vi "ControllerModels.vi"(9 "Gain in":dbl(slide)=3.0 scale=0.0..10.0, 10 "B":dbl, 11 "A":dbl) -> (3 "Plots":T1={"OpenLoop"=bytes[0], "Gain out"=bytes[146], "CL TF"=bytes[562], "Step Response Graph"=[{"time"=array[396 elements], array[396 elements]}], "Root Locus Graph"=[{[-13.1543317764195, -13.1543317764195], [27.765972114103178, -27.765972114103178]}, {[-26.308663552838997, 0.0], [0.0, 0.0]}, {[], []}, {[-13.154331776419498], [0.0]}, {array[551 elements], array[551 elements]}, {array[551 elements], array[551 elements]}], "Bode Magnitude"=[{"W"=[1.0, 1.0974987654930561, 1.2045035402587823, 1.3219411484660293, 1.45082877849594, 1.5922827933410926, 1.747528400007684, 1.9179102616724888, 2.104904144512021, 2.31012970008316, 2.5353644939701123, 2.7825594022071254, 3.0538555088334163, 3.351602650938843, 3.6783797718286344, 4.037017258596555, 4.430621457583881, 4.862601580065355, 5.33669923120631, 5.857020818056667, 6.428073117284322, 7.054802310718645, 7.742636826811273, 8.497534359086446, 9.326033468832202, 10.235310218990266, 11.23324032978028, 12.328467394420668, 13.530477745798079, 14.84968262254466, 16.297508346206453, 17.88649529057436, 19.63040650040272, 21.54434690031885, 23.644894126454087, 25.950242113997376, 28.480358684358034, 30.996999999999996, 31.257158496882383, 34.30469286314921, 37.64935806792471, 41.3201240011534, 45.34878508128586, 49.77023564332115, 54.62277217684346, 59.94842503189415, 60.99399999999999, 65.79332246575686, 72.20809018385471, 79.2482898353918, 86.97490026177842, 90.99099999999999, 95.4548456661835, 104.76157527896659, 114.9756995397737, 120.98799999999999, 126.18568830660217, 138.48863713938746, 151.99110829529354, 166.81005372000607, 183.07382802953703, 200.92330025650494, 220.51307399030483, 242.0128264794385, 265.608778294669, 291.50530628251806, 319.9267137797388, 351.11917342151366, 385.3528593710535, 422.9242874389505, 464.1588833612786, 509.4138014816387, 559.0810182512232, 613.5907273413183, 673.4150657750832, 739.0722033525791, 811.1308307896885, 890.2150854450401, 977.009957299227, 1072.2672220103252, 1176.8119524350006, 1291.5496650148864, 1417.474162926808, 1555.676143930475, 1707.3526474706944, 1873.8174228603882, 2056.512308348656, 2257.019719633925, 2477.0763559917164, 2718.5882427329466, 2983.6472402833456, 3274.5491628777354, 3593.813663804635, 3944.206059437664, 4328.761281083068, 4750.810162102807, 5214.008287999697, 5722.3676593502305, 6280.291441834267, 6892.612104349713, 7564.633275546306, 8302.175681319764, 9111.627561154914, 9850.015, 9880.011999999999, 9910.009, 9940.006, 9970.003, 10000.0], "Magnitude"=[21.548636949473586, 20.73927500165776, 19.929651557824194, 19.11971336672161, 18.309396388351143, 17.498623633018006, 16.687302578708522, 15.875322089526897, 15.062548746050313, 14.248822485839948, 13.433951439523174, 12.617705835762616, 11.799810838523417, 10.979938174582589, 10.157696411487612, 9.332619760848527, 8.50415531539156, 7.671648689191757, 6.834328129878358, 5.991287322571938, 5.141467322574313, 4.283638351698576, 3.4163825818107636, 2.5380795085862036, 1.6468960691316519, 0.7407842280817111, -0.18251074700562792, -1.1254278268777975, -2.0905502326886856, -3.080545366636483, -4.09808373757126, -5.145738487076201, -6.22587038275987, -7.34050665870406, -8.491225069395403, -9.679056063739079, -10.904415317281927, -12.052133376541043, -12.167075717542861, -13.466182727238525, -14.800310962512395, -16.167554244285633, -17.565637559869515, -18.99203797156701, -20.44410246107228, -21.919153353577915, -22.195621892315387, -23.414575415047665, -24.927882116358496, -26.45676133351209, -27.999102649045952, -28.7517404072417, -29.553009443353382, -31.116799279999533, -32.68899591767903, -33.55345326514365, -34.26831583311646, -35.85365157813415, -37.44405373043637, -39.03871269403542, -40.63694118912204, -42.23815794727944, -43.84187288830165, -45.447673885922754, -47.055215116635836, -48.664206914716885, -50.27440701592649, -51.885613052881716, -53.49765615972548, -55.11039554730617, -56.72371391895064, -58.33751360854884, -59.95171333539443, -61.566245482977166, -63.18105382105762, -64.79609160152121, -66.411319968546, -68.02670663248814, -69.64222476462781, -71.25785207660383, -72.87357005409736, -74.48936331920955, -76.10521910012109, -77.7211267901214, -79.33707758104266, -80.95306415861016, -82.56908044929585, -84.18512140999957, -85.80118285333359, -87.41726130249845, -89.03335387074826, -90.64945816128642, -92.26557218413345, -93.8816942870929, -95.49782309842678, -97.11395747925582, -98.73009648403611, -100.34623932774227, -101.96238535861991, -103.57853403556248, -105.19468490932783, -106.81083760694315, -108.42699181875705, -109.78062388444818, -109.83344690505376, -109.88610979208885, -109.93861351350975, -109.99095902852282, -110.04314728768948]}], "Bode Phase"=[{"W"=[1.0, 1.0974987654930561, 1.2045035402587823, 1.3219411484660293, 1.45082877849594, 1.5922827933410926, 1.747528400007684, 1.9179102616724888, 2.104904144512021, 2.31012970008316, 2.5353644939701123, 2.7825594022071254, 3.0538555088334163, 3.351602650938843, 3.6783797718286344, 4.037017258596555, 4.430621457583881, 4.862601580065355, 5.33669923120631, 5.857020818056667, 6.428073117284322, 7.054802310718645, 7.742636826811273, 8.497534359086446, 9.326033468832202, 10.235310218990266, 11.23324032978028, 12.328467394420668, 13.530477745798079, 14.84968262254466, 16.297508346206453, 17.88649529057436, 19.63040650040272, 21.54434690031885, 23.644894126454087, 25.950242113997376, 28.480358684358034, 30.996999999999996, 31.257158496882383, 34.30469286314921, 37.64935806792471, 41.3201240011534, 45.34878508128586, 49.77023564332115, 54.62277217684346, 59.94842503189415, 60.99399999999999, 65.79332246575686, 72.20809018385471, 79.2482898353918, 86.97490026177842, 90.99099999999999, 95.4548456661835, 104.76157527896659, 114.9756995397737, 120.98799999999999, 126.18568830660217, 138.48863713938746, 151.99110829529354, 166.81005372000607, 183.07382802953703, 200.92330025650494, 220.51307399030483, 242.0128264794385, 265.608778294669, 291.50530628251806, 319.9267137797388, 351.11917342151366, 385.3528593710535, 422.9242874389505, 464.1588833612786, 509.4138014816387, 559.0810182512232, 613.5907273413183, 673.4150657750832, 739.0722033525791, 811.1308307896885, 890.2150854450401, 977.009957299227, 1072.2672220103252, 1176.8119524350006, 1291.5496650148864, 1417.474162926808, 1555.676143930475, 1707.3526474706944, 1873.8174228603882, 2056.512308348656, 2257.019719633925, 2477.0763559917164, 2718.5882427329466, 2983.6472402833456, 3274.5491628777354, 3593.813663804635, 3944.206059437664, 4328.761281083068, 4750.810162102807, 5214.008287999697, 5722.3676593502305, 6280.291441834267, 6892.612104349713, 7564.633275546306, 8302.175681319764, 9111.627561154914, 9850.015, 9880.011999999999, 9910.009, 9940.006, 9970.003, 10000.0], "Magnitude"=[-92.17678142346449, -92.38877997223014, -92.6213725979796, -92.87654295647285, -93.15646034545647, -93.46349533053696, -93.80023611272149, -94.16950546680309, -94.57437798981827, -95.01819727935666, -95.50459250462488, -96.03749362942347, -96.62114428472908, -97.26011095750057, -97.95928674966291, -98.72388745665894, -99.55943711294196, -100.4717394564728, -101.46683099709112, -102.55091058395715, -103.73023964683034, -105.01100678610116, -106.39915033608405, -107.90013324436725, -109.5186665041156, -111.25838090695117, -113.1214524792275, -115.10819486002784, -117.21664188268032, -119.44215483057083, -121.77709940591497, -124.21064456282552, -126.72873561682742, -129.31428439086773, -131.94759821305436, -134.6070389635102, -137.26986825534652, -139.67711121214242, -139.91320311336142, -142.51498644913173, -145.05487387900345, -147.51495379057863, -149.8802466462038, -152.13896451642023, -154.28254447000393, -156.3054935723728, -156.66791790400825, -158.20509619577578, -159.9810367362953, -161.63498538015799, -163.17018468233277, -163.87357885445448, -164.59106346269309, -165.90289403326298, -167.11150020655438, -167.7320951166162, -168.22301727191194, -169.24370102687644, -170.1797806225077, -171.03734896234587, -171.82228425580317, -172.5401967217792, -173.19639511256148, -173.7958685091861, -174.3432796199893, -174.84296653383095, -175.2989505100373, -175.71494792015528, -176.09438489544456, -176.44041358795303, -176.7559292337515, -177.04358742648176, -177.30582117902247, -177.5448574806705, -177.76273315514678, -177.96130989787076, -178.1422884248995, -178.30722170515932, -178.45752727561646, -178.59449865858912, -178.71931591360948, -178.83305536474165, -178.93669854928976, -179.03114043633983, -179.11719696428358, -179.19561194590997, -179.26706338821853, -179.3321692721107, -179.39149283476124, -179.44554739492872, -179.49480075883878, -179.53967924165408, -179.58057133697895, -179.61783106437912, -179.65178102254643, -179.68271517352068, -179.71090138130296, -179.73658372625738, -179.7599846149005, -179.7813067030132, -179.80073464847715, -179.81843670882358, -179.83456619718544, -179.84696756281477, -179.84743218697574, -179.84789399837788, -179.84835302248612, -179.84880928445875, -179.84926280915235]}], "Closed Loop"=[{"time"=array[396 elements], array[396 elements]}]})   [LabVIEW 2020]
uses:
  <vilib>/addons/Control Design/_Model Construction/Model Creation.llb/Model Creation SubVI/cd_Create Transfer Function Model.vi
  <vilib>/addons/Control Design/_Utility/Model Viewer.llb/Model Viewer SubVI/cd_Draw Transfer Function Equation (TF).vi
  <vilib>/addons/Control Design/_Model Interconnection/Model Interconnection.llb/Model Interconnection SubVI/cd_Unit Feedback (TF and TF).vi
  <vilib>/addons/Control Design/_Time Response Analysis/Time Response.llb/Time Response subVI/cd_Step Response (Transfer Function).vi
  <vilib>/addons/Control Design/_Dynamic Analysis/Dynamic Analysis.llb/Dynamic Analysis subVI/cd_Root Locus (Transfer Function).vi
  <vilib>/addons/Control Design/_Frequency Response Analysis/Frequency Response.llb/Frequency Response subVI/cd_Bode (Transfer Function).vi
  <vilib>/addons/Control Design/_Model Construction/NI_LinSys_Model Creation.lvlib
  <vilib>/addons/Control Design/_Utility/NI_CD_Model Viewer.lvlib
  <vilib>/addons/Control Design/_Time Response Analysis/NI_CD_Time Response.lvlib
  <vilib>/addons/Control Design/_Dynamic Analysis/NI_CD_Dynamic Analysis.lvlib
  <vilib>/addons/Control Design/_Frequency Response Analysis/NI_CD_Frequency Response.lvlib
  <vilib>/addons/Control Design/_Model Interconnection/NI_CD_Model Interconnection.lvlib
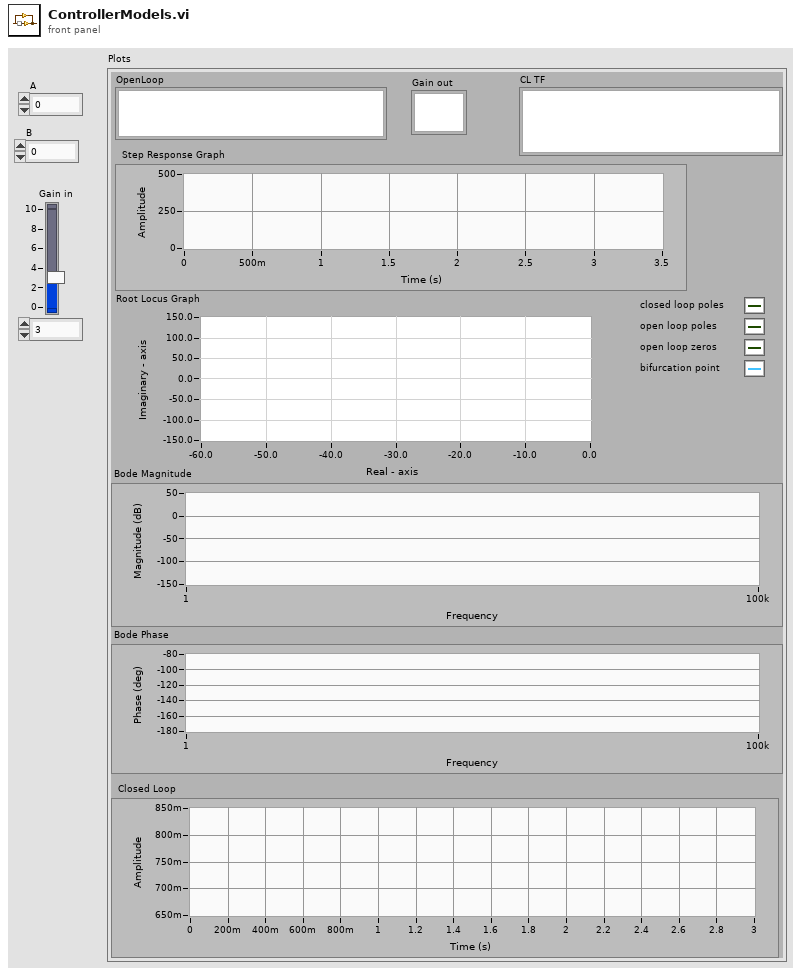
[diagram p1: front panel]
types:
  T1 = cluster{"OpenLoop":picture, "Gain out":picture, "CL TF":picture, "Step Response Graph":cluster{"time":dbl[], dbl[]}[], "Root Locus Graph":cluster{dbl[], dbl[]}[], "Bode Magnitude":cluster{"W":dbl[], "Magnitude":dbl[]}[], "Bode Phase":cluster{"W":dbl[], "Magnitude":dbl[]}[], "Closed Loop":cluster{"time":dbl[], dbl[]}[]}
  T2 = typedef "NI_LinSys_Model Typedefs.lvlib/CD Transfer Function Model (MIMO).ctl" = cluster{"properties":T3, "transfer function(s)":T4[][]}
  T3 = typedef "NI_LinSys_Model Typedefs.lvlib/CD General Elements.ctl" = cluster{"Model name":string, "Input names":string[], "Output names":string[], "Input Delays":dbl[], "Output Delays":dbl[], "Sampling Time":dbl, "Notes":string}
  T4 = typedef "NI_LinSys_Model Typedefs.lvlib/CD Transfer Function Model (SISO).ctl" = cluster{"Numerator":dbl[], "Denominator":dbl[], "delay":dbl}
  T5 = cluster{"Equation":picture, "Equation":picture, "Equation":picture, "Step Response Graph":cluster{"time":dbl[], dbl[]}[], "Root Locus Graph":cluster{dbl[], dbl[]}[], "Bode Magnitude":cluster{"W":dbl[], "Magnitude":dbl[]}[], "Bode Phase":cluster{"W":dbl[], "Magnitude":dbl[]}[], "Step Response Graph":cluster{"time":dbl[], dbl[]}[]}
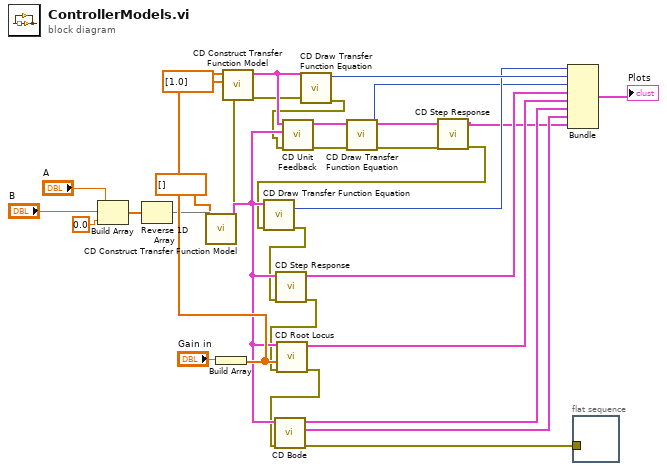
[diagram p0: block diagram]
diagram:
  n1 = Build Array("A", "B", 0.0 ("Numeric")) -> (w21:dbl[])
  n2 = Reverse 1D Array(array=w21) -> (reversed array=w23:dbl[])
  n3 = call-poly <vilib>:"CD Construct Transfer Function Model.vi"("Denominator"=w23, "Numerator"=dbl[] []) -> ("error out"=w10:errorcluster, "Transfer Function Model"=w25:T2)  [unwired: 8 in]
  n4 = Build Array("Gain in") -> (w26:dbl[])
  n5 = call-poly <vilib>:"CD Construct Transfer Function Model.vi"("error in (no error)"=w10, "Denominator"=dbl[] [1.0], "Numerator"=w26) -> ("error out"=w9:errorcluster, "Transfer Function Model"=w28:T2)  [unwired: 7 in]
  n6 = call-poly <vilib>:"CD Draw Transfer Function Equation.vi"("error in (no error)"=w9, "Transfer Function Model"=w28) -> ("error out"=w8:errorcluster, "Equation"=w19:picture)  [unwired: 7 in, 1 out]
  n7 = call-poly <vilib>:"CD Unit Feedback.vi"("error in (no error)"=w8, "Model 2"=w25, "Model 1"=w28) -> ("error out"=w7:errorcluster, "Closed-Loop Model"=w29:T2)  [unwired: 7 in]
  n8 = call-poly <vilib>:"CD Draw Transfer Function Equation.vi"("error in (no error)"=w7, "Transfer Function Model"=w29) -> ("error out"=w6:errorcluster, "Equation"=w17:picture)  [unwired: 7 in, 1 out]
  n9 = call-poly <vilib>:"CD Step Response.vi"("error in (no error)"=w6, "Transfer Function Model"=w29) -> ("error out"=w5:errorcluster, "Step Response Graph"=w11:cluster{"time":dbl[], dbl[]}[])  [unwired: 7 in, 1 out]
  n10 = call-poly <vilib>:"CD Draw Transfer Function Equation.vi"("error in (no error)"=w5, "Transfer Function Model"=w25) -> ("error out"=w4:errorcluster, "Equation"=w18:picture)  [unwired: 7 in, 1 out]
  n11 = call-poly <vilib>:"CD Step Response.vi"("error in (no error)"=w4, "Transfer Function Model"=w25) -> ("error out"=w3:errorcluster, "Step Response Graph"=w16:cluster{"time":dbl[], dbl[]}[])  [unwired: 7 in, 1 out]
  n12 = call-poly <vilib>:"CD Root Locus.vi"("error in (no error)"=w3, "Gain"=w26, "Transfer Function Model"=w25) -> ("error out"=w2:errorcluster, "Root Locus Graph"=w15:cluster{dbl[], dbl[]}[])  [unwired: 5 in, 2 out]
  n13 = call-poly <vilib>:"CD Bode.vi"("error in (no error)"=w2, "Transfer Function Model"=w25) -> ("error out"=w1:errorcluster, "Bode Phase"=w13:cluster{"W":dbl[], "Magnitude":dbl[]}[], "Bode Magnitude"=w14:cluster{"W":dbl[], "Magnitude":dbl[]}[])  [unwired: 5 in, 2 out]
  n14 = Bundle("Equation"=w18, "Equation"=w19, "Equation"=w17, "Step Response Graph"=w16, "Root Locus Graph"=w15, "Bode Magnitude"=w14, "Bode Phase"=w13, "Step Response Graph"=w11) -> (→"Plots":T5)  [unwired: 1 in]
  n15 = flat-sequence {
    tunnel: w1 -> [_]
    frame #0 {
    }
  }
